vi "REALTIME_TANK_PRESS.vi"() -> ()   [LabVIEW 2018]
uses:
  <vilib>/LabVIEW Targets/FPGA/cRIO/shared/nicrio_ModuleControls/nicrio_cRIO-9205_VoltageRange.ctl
  <vilib>/LabVIEW Targets/FPGA/cRIO/shared/nicrio_ModuleControls/nicrio_cRIO-9205_TerminalMode.ctl
  Pressure_Cluster.ctl
  Control_State.ctl
  <vilib>/rvi/Analysis/host/Private/Sample Rate To Loop Time (ticks).vi
  <vilib>/rvi/interface/RandomDataEmulation/nirviRandomDataOpen.vi
  <vilib>/rvi/interface/common/niFpgaCacheSessionInfoDynamic.vi
  <vilib>/Utility/error.llb/Error Cluster From Error Code.vi
  <vilib>/rvi/errors/niLvFpgaAdjustHostInterfaceError.vi
  <vilib>/FPGAPlugInAG/Dynamic/niLvFpga_Run_Dynamic.vi
  <vilib>/FPGAPlugInAG/Dynamic/niLvFpga_Close_Dynamic.vi
  <vilib>/rvi/interface/nirviOpenFPGA/nirviOpenFPGA.xnode
  FPGA_TANK_PRESS.vi
  <vilib>/rvi/interface/nirviReadWriteControl/nirviReadWriteControl.xnode
  <vilib>/rvi/interface/nirviMethod/nirviMethod.xnode
  <vilib>/rvi/interface/nirviCloseFPGA/nirviCloseFPGA.xnode
  <vilib>/rvi/interface/Simulation/niFpgaSimulationCallBeginRW.vi
  <vilib>/FPGAPlugInAG/Dynamic/niLvFpga_ReadFifo_Dynamic.vi
  <vilib>/rvi/errors/niLvFpgaMergeErrorWithErrorCode.vi
  NiFpgaLv.dll
  <vilib>/rvi/Analysis/host/Public/NI_FpgaMspHost.lvlib
panel:
  in  "Alarm Monitor":bool
  in  "Mod2/DO7":bool
  in  "Mod2/DO6":bool
  in  "Mod2/DO5":bool
  in  "Mod2/DO4":bool
  in  "Mod2/DO3":bool
  in  "Mod2/DO2":bool
  in  "Mod2/DO1":bool
  in  "Mod2/D00":bool
  in  "y":dbl
  in  "Pressure Cluster":T1
  out "element":string
  out "error out":errorcluster
  in  "stop":bool
  out "double precision float 2":dbl[][](array[numeric])
  out "Sample Rate [Hz]":dbl=10000.0 format="%#_6p"
  out "Elements Remaining":u32
  out "FPGA error out":errorcluster
  out "RT error out":errorcluster
  out "Voltage Input (V)":dbl[][](graph)
  out "Data FIFO Full":bool
  in  "AI Channel Settings":T4(array[cluster])=[{"Voltage Range"=enum."+/- 10V", "Terminal Mode"=enum."RSE"}, {"Voltage Range"=enum."+/- 10V", "Terminal Mode"=enum."RSE"}, {"Voltage Range"=enum."+/- 10V", "Terminal Mode"=enum."RSE"}, {"Voltage Range"=enum."+/- 10V", "Terminal Mode"=enum."RSE"}]
  in  "Target Acquisition Rate (Hz)":dbl=10000.0
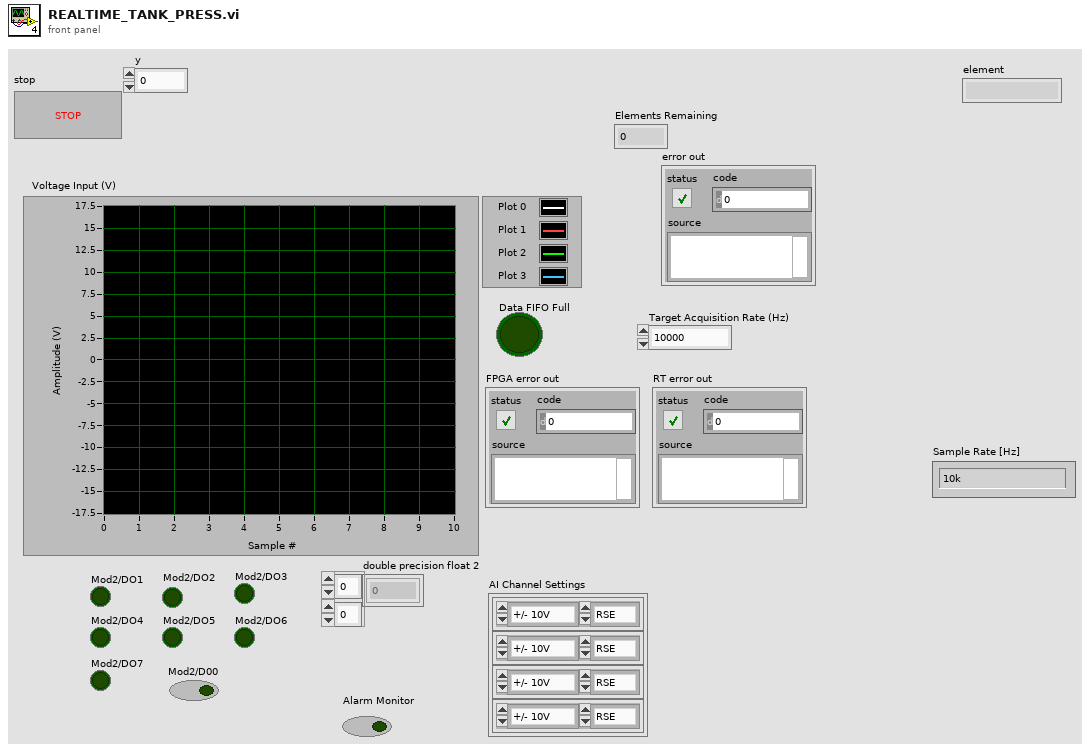
[diagram p1: front panel]
types:
  T1 = typedef "Pressure_Cluster.ctl" = cluster{"Pressure ENG1":dbl, "Pressure ENG2":dbl, "Pressure ENG3":dbl, "Pressure ENG4":dbl}
  T2 = typedef "nicrio_cRIO-9205_VoltageRange.ctl" = enum8{"+/- 10V", "+/- 5V", "+/- 1V", "+/- 200mV"}
  T3 = typedef "nicrio_cRIO-9205_TerminalMode.ctl" = enum8{"RSE", "NRSE", "DIFF"}
  T4 = cluster{"Voltage Range":T2, "Terminal Mode":T3}[]
  T5 = typedef "Control_State.ctl" = enum16{"Script", "Manual", "Safe", "Status"}
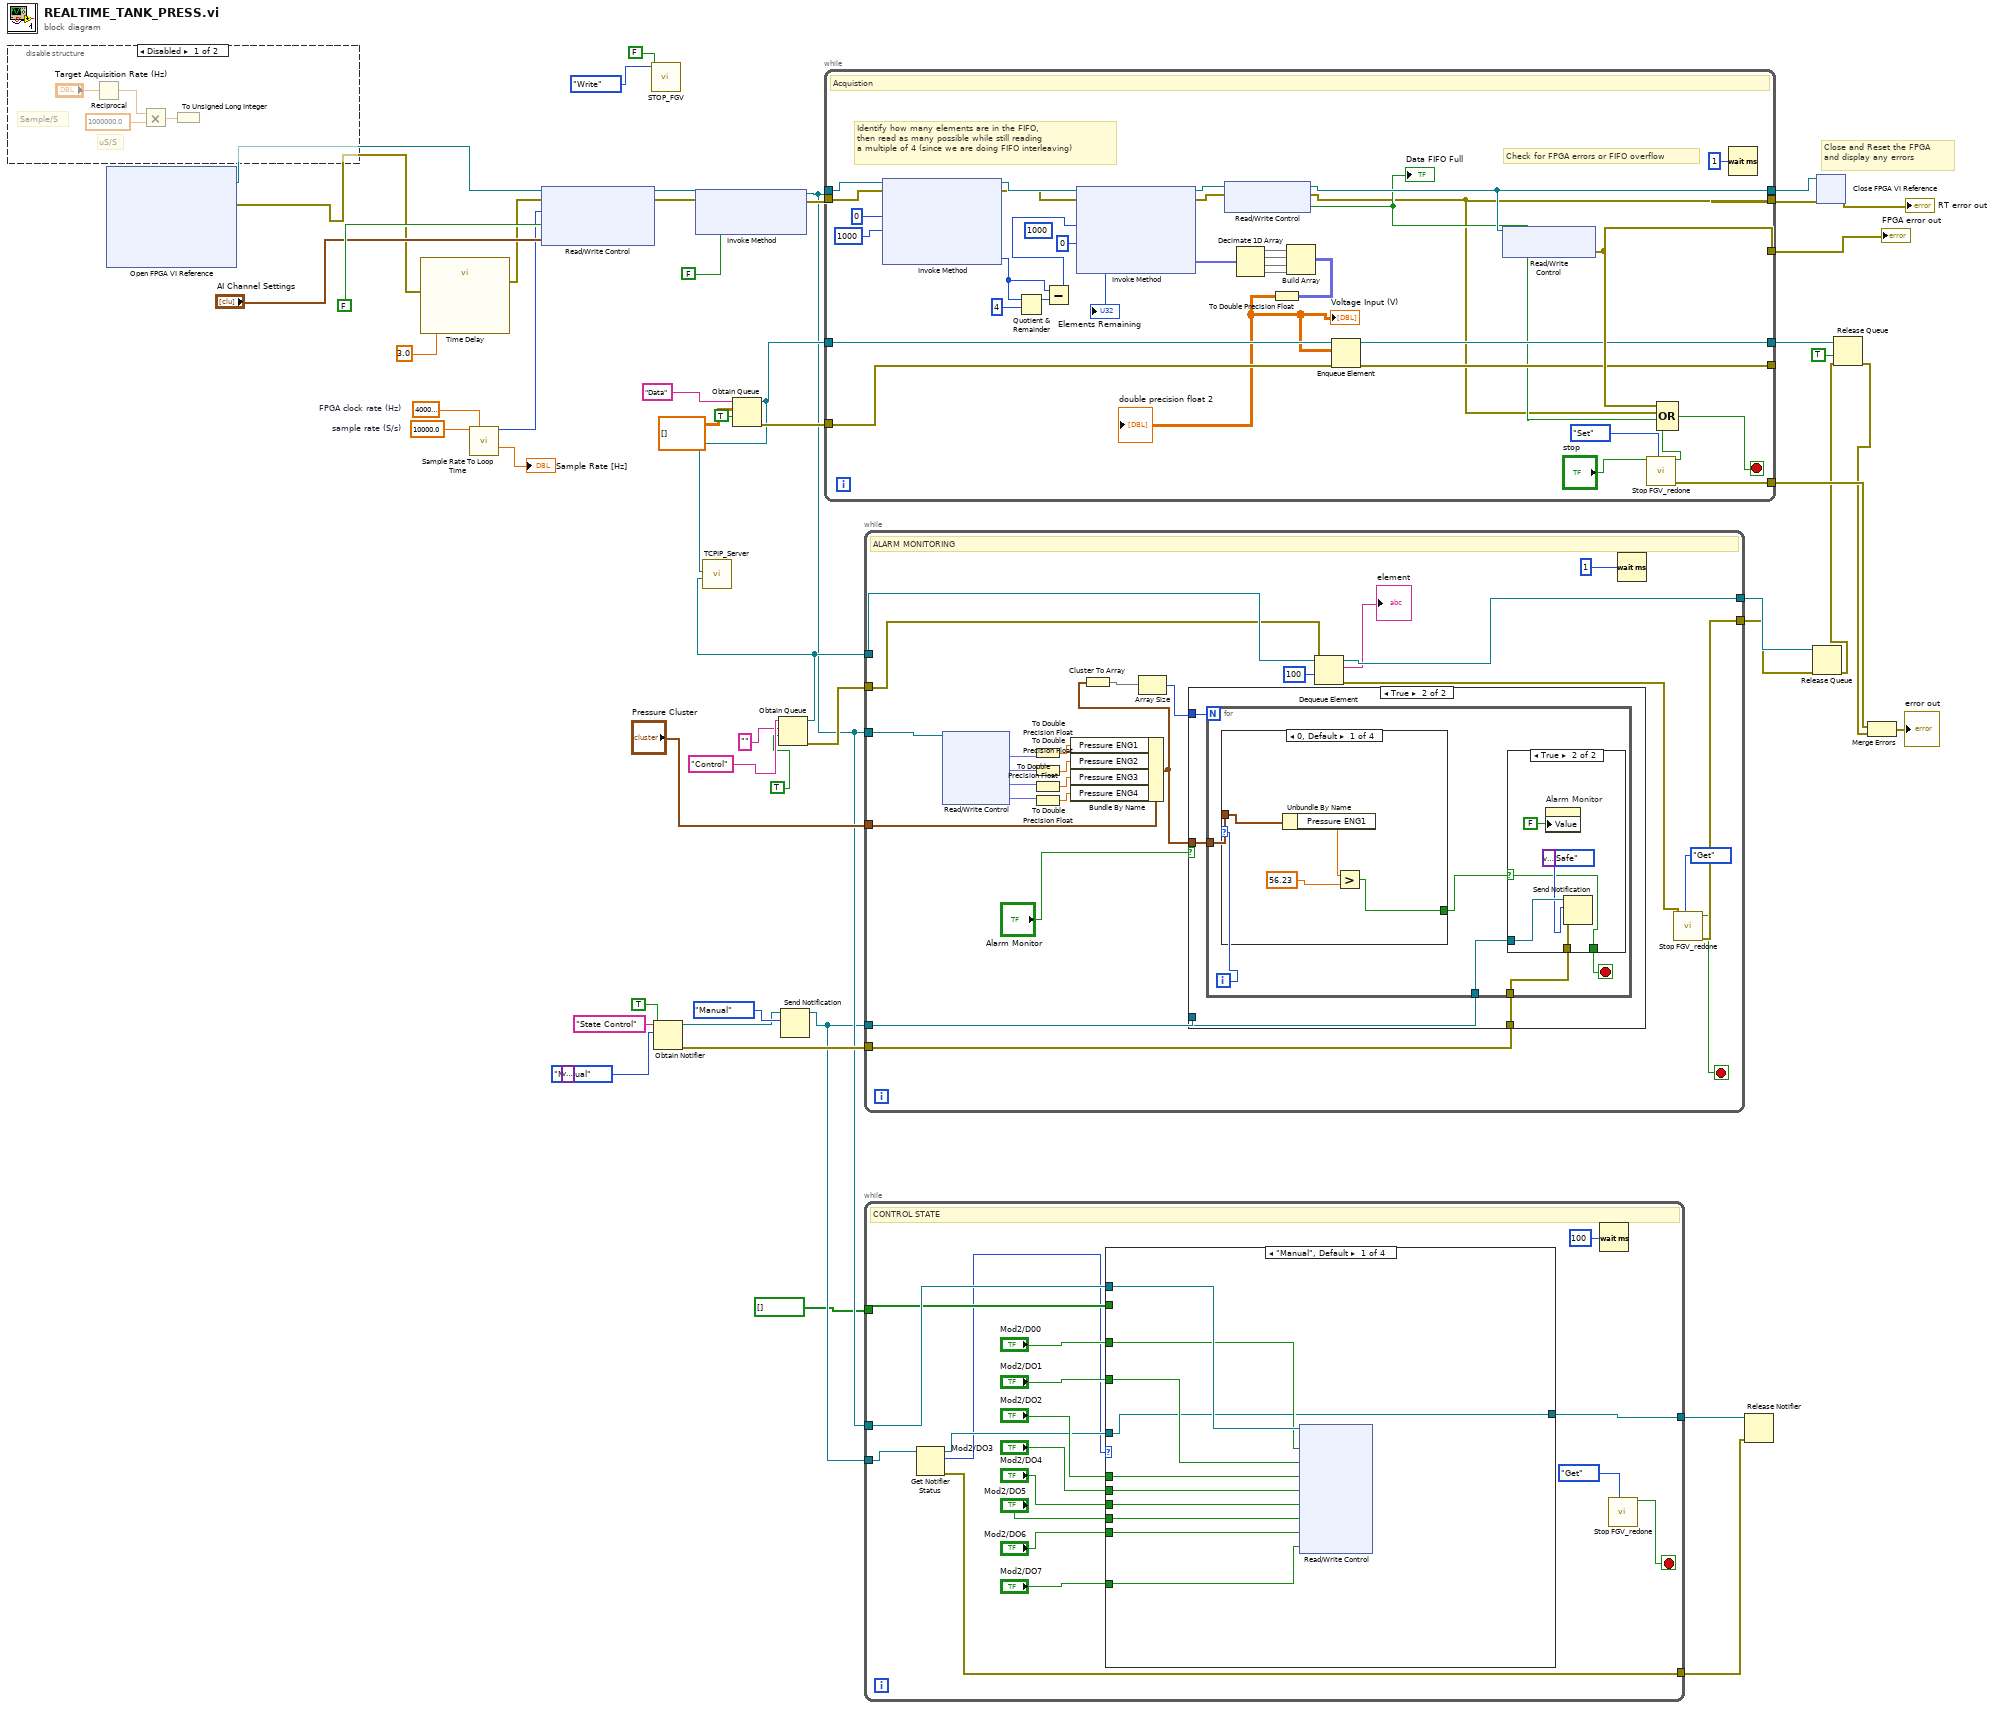
[diagram p0: block diagram]
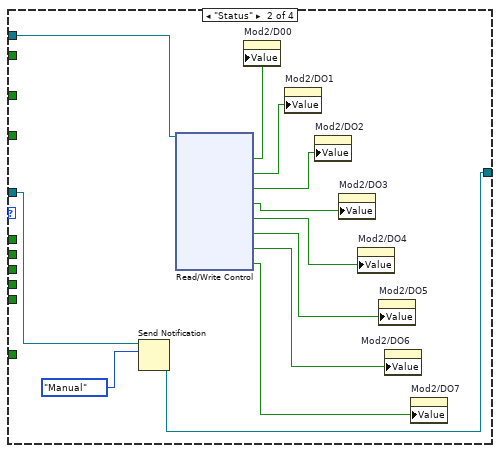
[diagram p2: hidden frame]
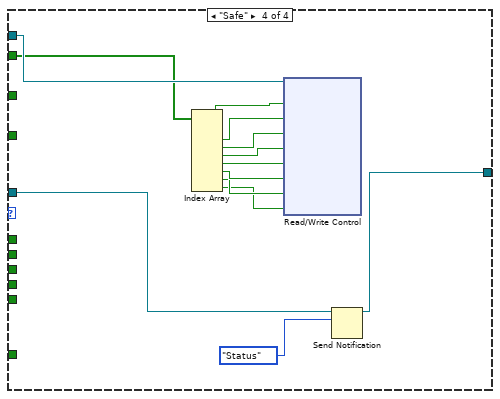
[diagram p4: hidden frame]
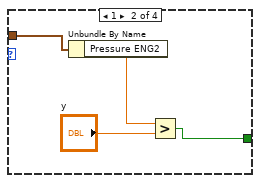
[diagram p7: hidden frame]
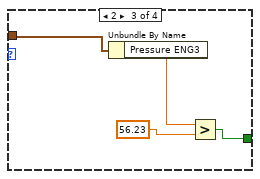
[diagram p8: hidden frame]
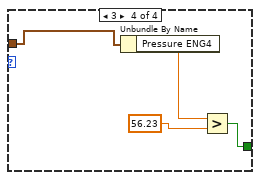
[diagram p9: hidden frame]
diagram:
  (unwired) variant ("element data type")
  w36 = 10000.0  # sample rate (S/s)
  w37 = 40000000.0  # FPGA clock rate (Hz)
  # "Close and Reset the FPGA\nand display any errors"
  n1 = disable-structure shown="Disabled" {
    frame Disabled {
      # "Sample/S"
      # "uS/S"
      n2 = Reciprocal(x="Target Acquisition Rate (Hz)") -> (1/x=w53:dbl)
      n3 = Multiply(x=w53, y=1000000.0) -> (x*y=w51:dbl)
      n4 = To Unsigned Long Integer(number=w51) -> ()  [unwired: 1 out]
    }
    frame Enabled {
    }
  }
  n5 = xnode "Open FPGA VI Reference"() -> ("FPGA VI Reference Out"=w28:refnum<k20>, "error out"=w27:errorcluster)  [unwired: 2 in]
  n6 = call "Time Delay"("error in (no error)"=w27, "Delay Time (s)"=3.0) -> ("error out"=w43:errorcluster)  [unwired: 9 in]
  n7 = call-poly <vilib>:"Sample Rate To Loop Time.vi"("sample rate (S/s)"=w36, "FPGA clock rate (Hz)"=w37) -> ("count (ticks/S)"=w35:u32, "actual sample rate (S/s)"=→"Sample Rate [Hz]":dbl)  [unwired: 11 in, 1 out]
  n8 = xnode "Read/Write Control"("FPGA VI Reference In"=w28, "error in"=w43, "Loop Rate (uS)"=w35, "Update AI Settings"=FALSE, "AI Channel Settings"="AI Channel Settings") -> ("FPGA VI Reference Out"=w32:refnum<k20>, "error out"=w31:errorcluster)
  n9 = call "STOP_FGV.vi"("Input"=FALSE, "Enum"=enum16{"Read", "Write"}."Write") -> ()  [unwired: 9 in, 1 out]
  n10 = Obtain Notifier(name (unnamed)="State Control", notification data type=Control_State."Manual" ("Mode"), create if not found? (T)=TRUE) -> (notifier out=w3:refnum<notifier>, error out=w8:errorcluster)  [unwired: 1 in, 1 out]
  n11 = xnode "Invoke Method"("FPGA VI Reference In"=w32, "error in"=w31, "Wait Until Done (F)"=FALSE) -> ("FPGA VI Reference Out"=w5:refnum<k20>, "error out"=w30:errorcluster)
  n12 = Obtain Queue(name (unnamed)="Data", element data type=dbl[][] [] ("Measurements (ue)"), create if not found? (T)=TRUE) -> (queue out=w15:refnum<queue>, error out=w39:errorcluster)  [unwired: 2 in, 1 out]
  n13 = Obtain Queue(name (unnamed)="Control", element data type="", create if not found? (T)=TRUE) -> (queue out=w13:refnum<queue>, error out=w20:errorcluster)  [unwired: 2 in, 1 out]
  n14 = call "TCPIP_Server.vi"("Message from Client"=w13, "Data to TCPIP"=w15) -> ()  [unwired: 10 in]
  n15 = Send Notification(notification=Control_State."Manual" ("Mode"), notifier=w3) -> (notifier out=w2:refnum<notifier>)  [unwired: 1 in, 1 out]
  n16 = while {
    tunnel: w5 -> [w76]
    tunnel: w30 -> [w75]
    tunnel: [w67] -> w47
    tunnel: [w69] -> w46
    tunnel: [w89] -> w45
    tunnel: w39 -> [w87]
    tunnel: [w86] -> w38
    tunnel: [w85] -> _
    tunnel: w15 -> [w84]
    tunnel: [w55] -> w24
    stop <- w66 stop-if-true
    (unwired) 1000 ("Timeout (ms)")
    # "Identify how many elements are in the FIFO, \nthen read as many possible while still reading\na multiple of 4 (since we are doing FIFO interleaving)"
    # "Check for FPGA errors or FIFO overflow"
    # "Acquistion"
    n17 = xnode "Invoke Method"("FPGA VI Reference In"=w76, "error in"=w75, "Number of Elements"=u32 0, "Timeout (ms)"=1000) -> ("FPGA VI Reference Out"=w74:refnum<k20>, "error out"=w73:errorcluster, "Elements Remaining"=w81:u32)  [unwired: 1 out]
    n18 = Quotient & Remainder(x=w81, y=u32 4) -> (x-y*floor(x/y)=w80:u32)  [unwired: 1 out]
    n19 = Subtract(x=w81, y=w80) -> (x-y=w72:u32)
    n20 = xnode "Invoke Method"("FPGA VI Reference In"=w74, "error in"=w73, "Number of Elements"=w72, "Timeout (ms)"=0) -> ("FPGA VI Reference Out"=w71:refnum<k20>, "error out"=w70:errorcluster, "Data"=w65:fxp<+/-,25,5>[], "Elements Remaining"=→"Elements Remaining":u32)
    n21 = xnode "Read/Write Control"("FPGA VI Reference In"=w71, "error in"=w70) -> ("FPGA VI Reference Out"=w69:refnum<k20>, "error out"=w67:errorcluster, "Data FIFO Full"=w68:bool)
    "Data FIFO Full" <- w68
    n22 = Decimate 1D Array(w65) -> (w64:fxp<+/-,25,5>[], w63:fxp<+/-,25,5>[], w62:fxp<+/-,25,5>[], w61:fxp<+/-,25,5>[])
    n23 = Build Array(w64, w63, w62, w61) -> (w60:fxp<+/-,25,5>[][])
    n24 = To Double Precision Float(number=w60) -> (double precision float=w59:dbl[][])
    "Voltage Input (V)" <- w59
    "double precision float 2" <- w59
    n25 = Enqueue Element(queue=w84, element=w59, error in (no error)=w87) -> (queue out=w86:refnum<queue>, error out=w85:errorcluster)  [unwired: 1 in, 1 out]
    n26 = xnode "Read/Write Control"("FPGA VI Reference In"=w69) -> ("FPGA Error Out"=w89:errorcluster)  [unwired: 1 in, 2 out]
    n27 = call "Stop FGV_redone.vi"("Mode"=enum16{"Set", "Get"}."Set", "Set Value"="stop") -> ("Error Out"=w55:errorcluster, "Get Value"=w57:bool)  [unwired: 8 in]
    n28 = Compound Arithmetic op=OR(w89, w67, w68, w57) -> (w66:bool)
    n29 = Wait (ms)(milliseconds to wait=u32 1 ("millisecond multiple")) -> ()  [unwired: 1 out]
  }
  "FPGA error out" <- w45
  n30 = while {
    tunnel: w13 -> [w113]
    tunnel: [w112] -> w19
    tunnel: [w114] -> w18
    tunnel: w20 -> [w110]
    tunnel: w5 -> [w105]
    tunnel: w2 -> [w91]
    tunnel: "Pressure Cluster" -> [w96]
    tunnel: w8 -> [w92]
    stop <- w108 stop-if-true
    # "ALARM MONITORING"
    n31 = xnode "Read/Write Control"("FPGA VI Reference In"=w105) -> ("Mod1/AI0"=w104:fxp<+/-,26,5>, "Mod1/AI1"=w103:fxp<+/-,26,5>, "Mod1/AI2"=w102:fxp<+/-,26,5>, "Mod1/AI3"=w101:fxp<+/-,26,5>)  [unwired: 1 in, 2 out]
    n32 = To Double Precision Float(number=w104) -> (double precision float=w100:dbl)
    n33 = To Double Precision Float(number=w103) -> (double precision float=w99:dbl)
    n34 = To Double Precision Float(number=w102) -> (double precision float=w98:dbl)
    n35 = To Double Precision Float(number=w101) -> (double precision float=w97:dbl)
    n36 = Bundle By Name(cluster=w96, "Pressure ENG1"=w100, "Pressure ENG2"=w99, "Pressure ENG3"=w98, "Pressure ENG4"=w97) -> (w95:T1)
    n37 = Cluster To Array(cluster=w95) -> (array=w94:dbl[])
    n38 = Array Size(array=w94) -> (size(s)=w93:i32)
    n39 = case shown="True" "Alarm Monitor" {
      tunnel: w95 -> [_ w119]
      tunnel: w93 -> [_ w118]
      tunnel: w92 -> [_ w117]
      tunnel: w91 -> [_ w116]
      frame False {
      }
      frame True {
        n40 = for {
          N: w118 -> [_]
          tunnel: w119 -> [w125]
          tunnel: w116 -> [w123]
          tunnel: w117 -> [w122]
          i -> [w124]
          stop <- w120 stop-if-true
          n41 = case shown="0, Default" w124 {
            tunnel: w125 -> [w135 w139 w142 w146]
            tunnel: [w132 w137 w140 w144] -> w121
            frame 0, Default {
              n42 = Unbundle By Name(w135) -> ("Pressure ENG1"=w133:dbl)
              n43 = Greater?(x=w133, y=56.23) -> (0:w132:bool)
            }
            frame 1 {
              n44 = Unbundle By Name(w139) -> ("Pressure ENG2"=w138:dbl)
              n45 = Greater?(x=w138, y="y") -> (0:w137:bool)
            }
            frame 2 {
              n46 = Unbundle By Name(w142) -> ("Pressure ENG3"=w143:dbl)
              n47 = Greater?(x=w143, y=56.23) -> (0:w140:bool)
            }
            frame 3 {
              n48 = Unbundle By Name(w146) -> ("Pressure ENG4"=w147:dbl)
              n49 = Greater?(x=w147, y=56.23) -> (0:w144:bool)
            }
          }
          n50 = case shown="True" w121 {
            selector: w121 -> [w126 w128]
            tunnel: w123 -> [_ w131]
            tunnel: w122 -> [_ w129]
            tunnel: [w126 w128] -> w120
            frame False {
            }
            frame True {
              (unwired) variant ("element data type")
              n51 = property on="Alarm Monitor" class="Bool (strict)"("Value"=FALSE ("reset")) -> ()  [unwired: 2 in, 2 out]
              n52 = Send Notification(notification=Control_State."Safe" ("Mode"), notifier=w131, error in (no error)=w129) -> ()  [unwired: 2 out]
            }
          }
        }
      }
    }
    n53 = Dequeue Element(queue=w113, timeout in ms (-1)=100, error in (no error)=w110) -> (queue out=w112:refnum<queue>, element=→"element":string, error out=w111:errorcluster)  [unwired: 1 out]
    n54 = Wait (ms)(milliseconds to wait=u32 1 ("millisecond multiple")) -> ()  [unwired: 1 out]
    n55 = call "Stop FGV_redone.vi"("Mode"=enum16{"Set", "Get"}."Get", "Error In"=w111) -> ("Error Out"=w114:errorcluster, "Get Value"=w108:bool)  [unwired: 8 in]
  }
  n56 = while {
    tunnel: w2 -> [w162]
    tunnel: [w149] -> w7
    tunnel: [w161] -> w6
    tunnel: w5 -> [w160]
    tunnel: bool[] [] -> [w159]
    stop <- w163 stop-if-true
    # "CONTROL STATE"
    n57 = Get Notifier Status(notifier=w162) -> (notifier out=w150:refnum<notifier>, current notification=w148:T5, error out=w161:errorcluster)  [unwired: 1 in, 2 out]
    n58 = case shown="\"Manual\", Default" w148 {
      tunnel: w159 -> [_ _ _ w192]
      tunnel: w160 -> [w175 w179 _ w193]
      tunnel: "Mod2/D00" -> [w174 _ _ _]
      tunnel: "Mod2/DO1" -> [w173 _ _ _]
      tunnel: "Mod2/DO2" -> [w172 _ _ _]
      tunnel: "Mod2/DO3" -> [w171 _ _ _]
      tunnel: "Mod2/DO4" -> [w170 _ _ _]
      tunnel: "Mod2/DO5" -> [w169 _ _ _]
      tunnel: "Mod2/DO6" -> [w168 _ _ _]
      tunnel: "Mod2/DO7" -> [w167 _ _ _]
      tunnel: w150 -> [w166 w178 w188 w191]
      tunnel: [w166 w176 w188 w190] -> w149
      frame "Manual", Default {
        n59 = xnode "Read/Write Control"("FPGA VI Reference In"=w175, "Mod2/DO0"=w174, "Mod2/DO1"=w173, "Mod2/DO2"=w172, "Mod2/DO3"=w171, "Mod2/DO4"=w170, "Mod2/DO5"=w169, "Mod2/DO6"=w168, "Mod2/DO7"=w167) -> ()  [unwired: 1 in, 2 out]
      }
      frame "Status" {
        n60 = Send Notification(notification=Control_State."Manual" ("Mode"), notifier=w178) -> (notifier out=w176:refnum<notifier>)  [unwired: 1 in, 1 out]
        n61 = xnode "Read/Write Control"("FPGA VI Reference In"=w179) -> ("Mod2/DO0"=w187:bool, "Mod2/DO1"=w186:bool, "Mod2/DO2"=w185:bool, "Mod2/DO3"=w184:bool, "Mod2/DO4"=w183:bool, "Mod2/DO5"=w182:bool, "Mod2/DO6"=w181:bool, "Mod2/DO7"=w180:bool)  [unwired: 1 in, 2 out]
        n62 = property on="Mod2/D00" class="Bool (strict)"("Value"=w187) -> ()  [unwired: 2 in, 2 out]
        n63 = property on="Mod2/DO1" class="Bool (strict)"("Value"=w186) -> ()  [unwired: 2 in, 2 out]
        n64 = property on="Mod2/DO2" class="Bool (strict)"("Value"=w185) -> ()  [unwired: 2 in, 2 out]
        n65 = property on="Mod2/DO3" class="Bool (strict)"("Value"=w184) -> ()  [unwired: 2 in, 2 out]
        n66 = property on="Mod2/DO4" class="Bool (strict)"("Value"=w183) -> ()  [unwired: 2 in, 2 out]
        n67 = property on="Mod2/DO5" class="Bool (strict)"("Value"=w182) -> ()  [unwired: 2 in, 2 out]
        n68 = property on="Mod2/DO6" class="Bool (strict)"("Value"=w181) -> ()  [unwired: 2 in, 2 out]
        n69 = property on="Mod2/DO7" class="Bool (strict)"("Value"=w180) -> ()  [unwired: 2 in, 2 out]
      }
      frame "Script" {
      }
      frame "Safe" {
        n70 = Index Array(array=w192) -> (element #1=w201:bool, element #2=w200:bool, element #3=w199:bool, element #4=w198:bool, element #5=w197:bool, element #6=w196:bool, element #7=w195:bool, element #8=w194:bool)  [unwired: 8 in]
        n71 = xnode "Read/Write Control"("FPGA VI Reference In"=w193, "Mod2/DO0"=w201, "Mod2/DO1"=w200, "Mod2/DO2"=w199, "Mod2/DO3"=w198, "Mod2/DO4"=w197, "Mod2/DO5"=w196, "Mod2/DO6"=w195, "Mod2/DO7"=w194) -> ()  [unwired: 1 in, 2 out]
        n72 = Send Notification(notification=Control_State."Status" ("Mode"), notifier=w191) -> (notifier out=w190:refnum<notifier>)  [unwired: 1 in, 1 out]
      }
    }
    n73 = Wait (ms)(milliseconds to wait=u32 100 ("millisecond multiple")) -> ()  [unwired: 1 out]
    n74 = call "Stop FGV_redone.vi"("Mode"=enum16{"Set", "Get"}."Get") -> ("Get Value"=w163:bool)  [unwired: 9 in, 1 out]
  }
  n75 = Release Notifier(notifier=w7, error in (no error)=w6) -> ()  [unwired: 1 in, 3 out]
  n76 = Release Queue(queue=w19, error in (no error)=w18) -> (error out=w16:errorcluster)  [unwired: 1 in, 2 out]
  n77 = xnode "Close FPGA VI Reference"("FPGA VI Reference In"=w46, "error in"=w47) -> ("error out"=→"RT error out":errorcluster)
  n78 = Release Queue(queue=w38, force destroy? (F)=TRUE, error in (no error)=w16) -> (error out=w17:errorcluster)  [unwired: 2 out]
  n79 = Merge Errors(w24, w17) -> (→"error out":errorcluster)
